vi "Alarma_Tolerancia_Voltaje_G5.vi"(7 "ID_EQUIPO":i32=1, 8 "AVG_VL_VL":sgl, 9 "V3_V1":sgl, 10 "V2_V3":sgl, 11 "V1_V2":sgl) -> (3 "alarm out":T1)   [LabVIEW 2018]
uses:
  Global/TimerReferences.vi
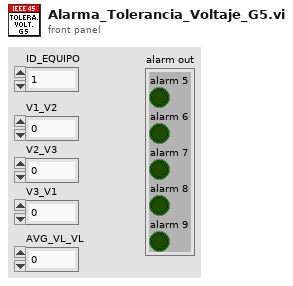
[diagram p1: front panel]
types:
  T1 = cluster{"alarm 5":bool, "alarm 6":bool, "alarm 7":bool, "alarm 8":bool, "alarm 9":bool}
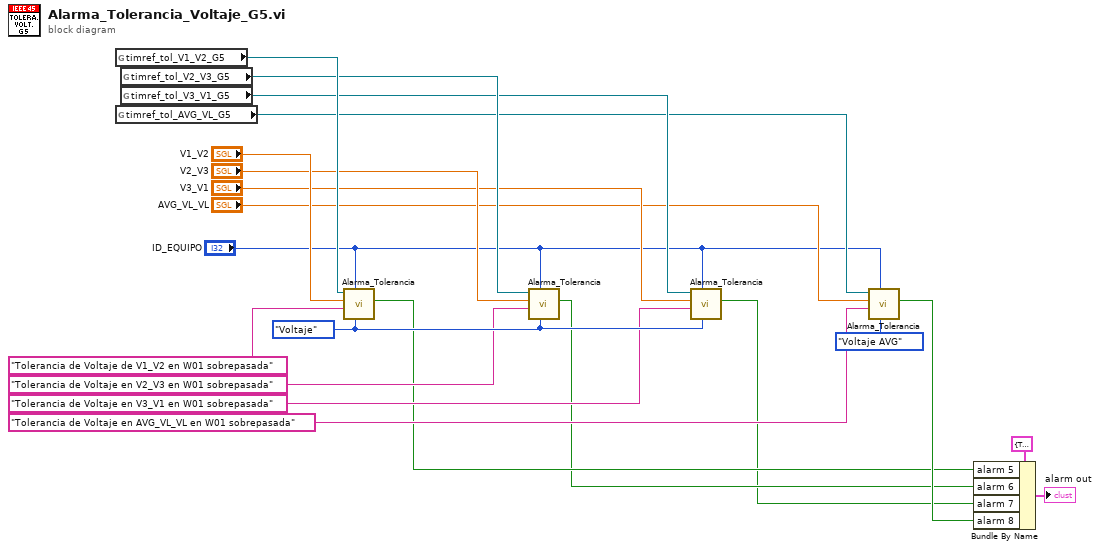
[diagram p0: block diagram]
diagram:
  w12 = enum16{"Voltaje", "Frecuencia", "Voltaje AVG"}."Voltaje" ("Tipo Señal")
  n1 = global read "TimerReferences.vi" "timref_tol_V1_V2_G5"() -> (w21:refnum<data-value>)
  n2 = global read "TimerReferences.vi" "timref_tol_AVG_VL_G5"() -> (w18:refnum<data-value>)
  n3 = global read "TimerReferences.vi" "timref_tol_V2_V3_G5"() -> (w20:refnum<data-value>)
  n4 = global read "TimerReferences.vi" "timref_tol_V3_V1_G5"() -> (w19:refnum<data-value>)
  n5 = call "Alarma_Tolerancia.vi"("Tipo Señal"=w12, "ID_EQUIPO"="ID_EQUIPO", "Motivo Alarma"="Tolerancia de Voltaje de V1_V2 en W01 sobrepasada", "Señal in"="V1_V2", "timref in"=w21) -> ("alarm"=w3:bool)  [unwired: 6 in]
  n6 = call "Alarma_Tolerancia.vi"("Tipo Señal"=w12, "ID_EQUIPO"="ID_EQUIPO", "Motivo Alarma"="Tolerancia de Voltaje en V2_V3 en W01 sobrepasada", "Señal in"="V2_V3", "timref in"=w20) -> ("alarm"=w2:bool)  [unwired: 6 in]
  n7 = call "Alarma_Tolerancia.vi"("Tipo Señal"=w12, "ID_EQUIPO"="ID_EQUIPO", "Motivo Alarma"="Tolerancia de Voltaje en V3_V1 en W01 sobrepasada", "Señal in"="V3_V1", "timref in"=w19) -> ("alarm"=w1:bool)  [unwired: 6 in]
  n8 = call "Alarma_Tolerancia.vi"("Tipo Señal"=enum16{"Voltaje", "Frecuencia", "Voltaje AVG"}."Voltaje AVG", "ID_EQUIPO"="ID_EQUIPO", "Motivo Alarma"="Tolerancia de Voltaje en AVG_VL_VL en W01 sobrepasada", "Señal in"="AVG_VL_VL", "timref in"=w18) -> ("alarm"=w4:bool)  [unwired: 6 in]
  n9 = Bundle By Name(cluster=T1 {"alarm 5"=TRUE, "alarm 6"=TRUE, "alarm 7"=TRUE, "alarm 8"=TRUE, "alarm 9"=TRUE}, "alarm 5"=w3, "alarm 6"=w2, "alarm 7"=w1, "alarm 8"=w4) -> (→"alarm out":T1)
